vi "PP Template (UserEvent).vi"() -> ()   [LabVIEW 2011, in "Messenging.lvlib" / "PP Template (UserEvent).lvclass"]
uses:
  PP Template (UserEvent).lvclass
  Interprocess Messenger/TextVarientMessage/MSG.lvclass
  Parallel Process.lvclass
  Interprocess Messenger/EventMessenger/EventMessenger.lvclass
  ObserverRegister/ObserverRegistry.lvclass
  Interprocess Messenger/TextVarientMessage/Write (no data).vi
  Interprocess Messenger/ErrorMessage/Write ErrorMessage.vi
  Interprocess Messenger/ErrorMessage/ErrorMessage.lvclass
  Interprocess Messenger/TextVarientMessage/Write VarMessage.vi
  Interprocess Messenger/VarMessage/VarMessage.lvclass
panel:
  out "date/time string":string
  in  "Startup Message":refnum<class "MSG.lvclass">
  # "EventMesssenger based"
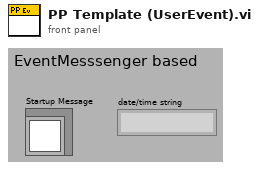
[diagram p1: front panel]
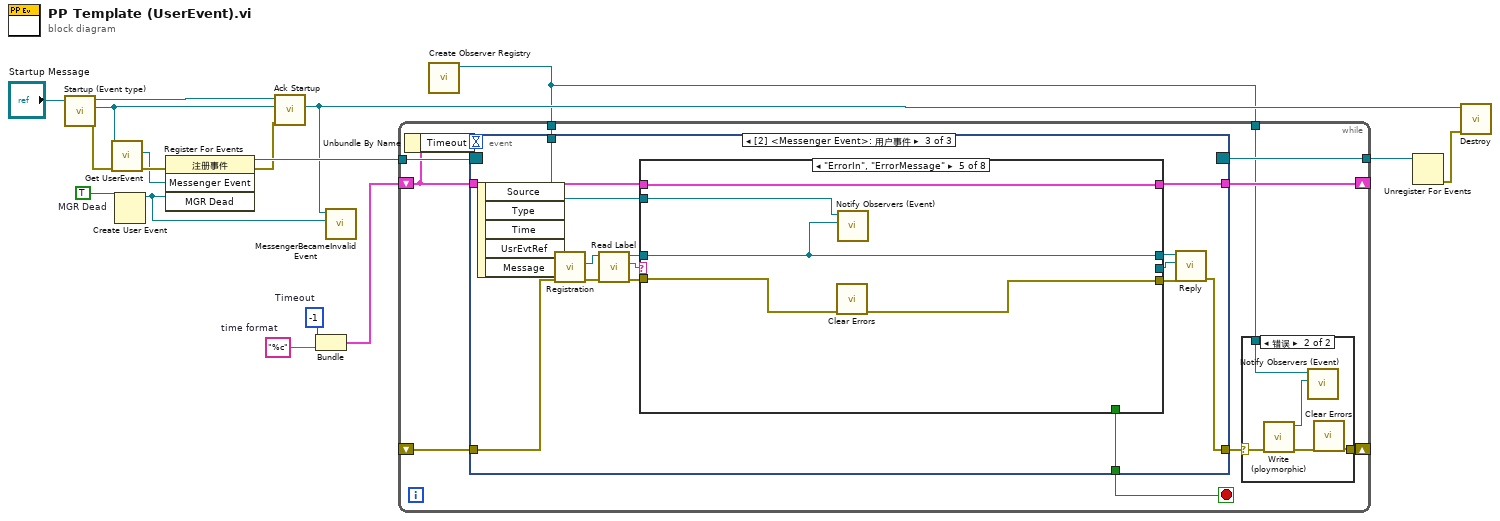
[diagram p0: block diagram]
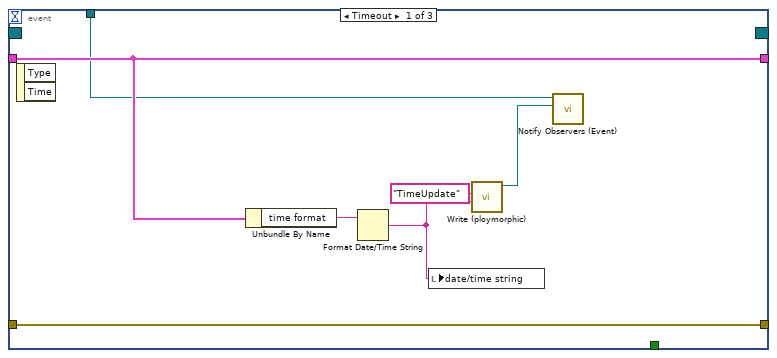
[diagram p3: hidden frame]
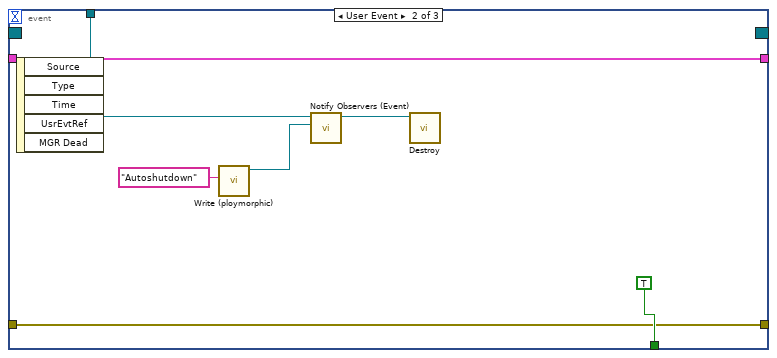
[diagram p4: hidden frame]
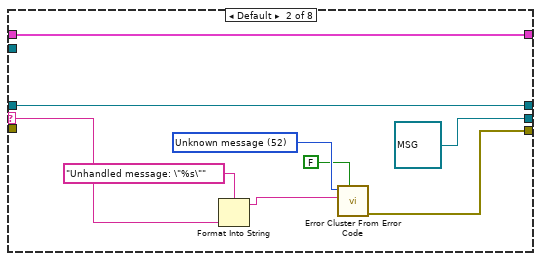
[diagram p6: hidden frame]
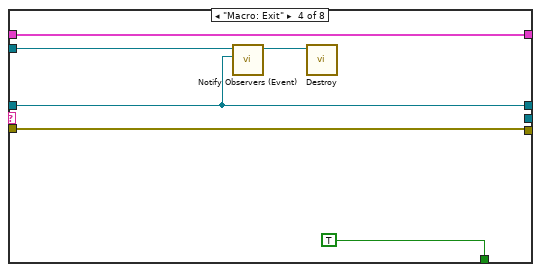
[diagram p8: hidden frame]
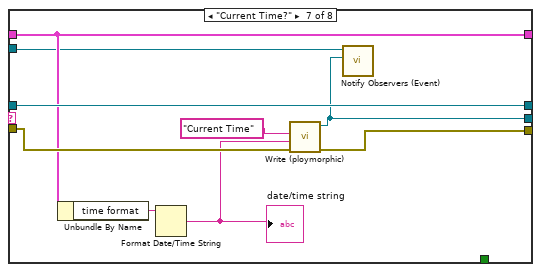
[diagram p10: hidden frame]
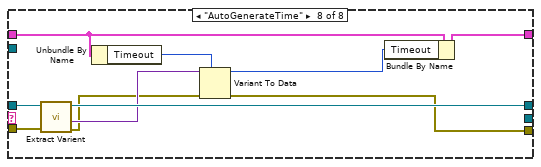
[diagram p11: hidden frame]
diagram:
  w2 = "%c"  # time format
  w6 = TRUE  # MGR Dead
  w9 = -1  # Timeout
  n1 = call "Startup (Event type).vi"("Startup Message"="Startup Message") -> ("error out"=w15:errorcluster, "Command Messenger out"=w17:refnum<class "EventMessenger.lvclass">, "Starup Message"=w16:refnum<class "MSG.lvclass">)  [unwired: 2 in, 6 out]
  n2 = call-dynamic "Get UserEvent.vi"("error in"=w15, "EventMessenger"=w17) -> ("error out"=w13:errorcluster, "Messenger Event"=w7:refnum<user-event>)  [unwired: 8 out]
  n3 = Create User Event(user event datatype=w6) -> (user event=w4:refnum<user-event>)  [unwired: 1 in, 1 out]
  n4 = register-events(error in=w13, w7, w4) -> (reference out=w12:refnum<event-registration>, error out=w5:errorcluster)  [unwired: 1 in]
  n5 = call "Ack Startup.vi"("error in"=w5, "Command Messenger"=w17, "Starup Message"=w16) -> ("Command Messenger"=w3:refnum<class "EventMessenger.lvclass">)  [unwired: 3 in, 5 out]
  n6 = Bundle("Timeout"=w9, "time format"=w2) -> (w8:cluster{"Timeout":i32, "time format":string})  [unwired: 1 out]
  n7 = call "MessengerBecameInvalid Event.vi"("MGR became Invalid"=w4, "Messenger"=w3) -> ()  [unwired: 1 in, 9 out]
  n8 = call "Create Observer Registry.vi"() -> ("ObsReg"=w1:refnum<class "ObserverRegistry.lvclass">)  [unwired: 1 in, 10 out]
  n9 = while {
    tunnel: w12 -> [w28]
    tunnel: [w27] -> w11
    shift-right: [w21] -> _
    shift-left: w8 -> [w25]
    shift-right: [w20] -> _
    shift-left: _ -> [w23]
    tunnel: w1 -> [w19]
    tunnel: w1 -> [w18]
    stop <- w26 stop-if-true
    n10 = Unbundle By Name(w25) -> ("Timeout"=w24:i32)
    n11 = event shown="[2] <Messenger Event>: 用户事件" {
      selector: w28 -> [_ _ _]
      dyn-events: [_ _ _] -> w27
      timeout: w24 -> [_ _ _]
      tunnel: [_ TRUE ("Shutdown if Receiver Dead") w54] -> w26
      tunnel: w25 -> [w37 w48 w56]
      tunnel: [w37 w48 w55] -> w21
      tunnel: [w35 w46 w53] -> w22
      tunnel: w23 -> [w35 w46 w52]
      tunnel: w19 -> [w36 w45 w49]
      event Timeout {
        n12 = event-data() -> ()  [unwired: 3 out]
        n13 = Unbundle By Name(w37) -> ("time format"=w41:string)
        n14 = Format Date/Time String(time format string (%c)=w41) -> (date/time string=w38:string)  [unwired: 2 out]
        n15 = local write "date/time string"(w38) -> ()
        n16 = call-poly "Write (ploymorphic).vi"("Varient"=w38, "Label"="TimeUpdate") -> ("Message"=w39:refnum<class "VarMessage.lvclass">)  [unwired: 1 in, 8 out]
        n17 = call "Notify Observers (Event).vi"("Message"=w39, "ObserverRegistry in"=w36) -> ()  [unwired: 1 in, 9 out]
      }
      event User Event {
        n18 = event-data() -> ()  [unwired: 6 out]
        n19 = call-poly "Write (ploymorphic).vi"("Label"="Autoshutdown") -> ("Message"=w42:refnum<class "MSG.lvclass">)  [unwired: 1 in, 9 out]
        n20 = call "Notify Observers (Event).vi"("Message"=w42, "ObserverRegistry in"=w45) -> ("ObserverRegistry out"=w44:refnum<class "ObserverRegistry.lvclass">)  [unwired: 1 in, 8 out]
        n21 = call "Destroy.vi"("ObserverRegistry.lvclass in"=w44) -> ()  [unwired: 1 in, 10 out]
      }
      event User Event {
        n22 = event-data() -> ("Message"=w51:refnum<class "MSG.lvclass">)  [unwired: 5 out]
        n23 = call "Registration.vi"("Message"=w51, "ObserverRegistry in"=w49) -> ("Message (Register Commands filtered out)"=w50:refnum<class "MSG.lvclass">)  [unwired: 1 in, 8 out]
        n24 = call-dynamic "Read Label.vi"("error in (no error)"=w52, "Message"=w50) -> ("error out"=w58:errorcluster, "Label"=w57:string, "Message"=w59:refnum<class "MSG.lvclass">)  [unwired: 7 out]
        n25 = case shown="\"ErrorIn\", \"ErrorMessage\"" w57 {
          selector: w57 -> [_ w74 _ _ _ _ _ _]
          tunnel: w58 -> [w65 _ w77 w79 w85 w91 w99 w108]
          tunnel: w59 -> [w64 w68 w76 w80 w87 w90 w100 w110]
          tunnel: [w65 w69 w77 w79 w84 w91 w98 w101] -> w62
          tunnel: [w64 w68 w76 w80 w87 w90 w100 w109] -> w60
          tunnel: [_ refnum<class "MSG.lvclass"> refnum ("Messenging.lvlib:Interprocess Message") _ _ _ _ w94 _] -> w61
          tunnel: [_ _ _ TRUE _ _ _ _] -> w54
          tunnel: [w63 w66 w75 w83 w88 w89 w97 w104] -> w55
          tunnel: w56 -> [w63 w66 w75 w83 w88 w89 w97 w106]
          tunnel: w49 -> [_ _ _ w78 w86 _ w93 _]
          frame "------- Core ----------" {
            # "Core Cases for template"
          }
          frame Default {
            w71 = 52 items=["No error", "Argument error", "Memory is full", "Out of zone", "End of file", "File already open", "Generic file I/O error", "File not found", "File permission error", "Disk is full", "Duplicate path", "Too many files open", "System feature not enabled", "Resource file not found", "Cannot add resource", "Resource not found", "Image not found", "Image memory error", "Pen does not exist", "Config type invalid", "Config token not found", "Config parse error", "Config memory error", "Bad external code format", "Bad external code offset", "External code not present", "Null window", "Destroy window error", "Null menu", "Print aborted", "Bad print record", "Print driver error", "Windows error during printing", "Memory error during printing", "Print dialog error", "Generic print error", "Invalid device refnum", "Device not found", "Device parameter error", "Device unit error", "Cannot open device", "Device call aborted", "Generic error", "Cancelled by user", "Object ID too low", "Object ID too high", "Object not in heap", "Unknown heap", "Unknown object (invalid DefProc)", "Unknown object (DefProc not in table)", "Message out of range", "Invalid (null) method", "Unknown message", "Manager call not supported", "Bad address", "Network operation in progress", "Network operation timed out", "Connection is busy", "Network attribute not supported", "Network error", "Address in use", "System out of memory", "Connection aborted", "Connection refused", "Not connected", "Already connected", "Connection closed", "Initialization error (interapplication manager)", "Bad occurrence", "Wait on unbound occurrence handler", "Occurrence queue overflow", "Datalog type conflict", "Unused", "Unrecognized type (interapplication manager)", "Memory corrupt", "Failed to make temporary DLL", "Old CIN version", "Drag socket not found", "Failed to load drop-object", "Failed to register OLE object", "Failed to release OLE object", "Format specifier type mismatch", "Unknown format specifier", "Too few format specifiers", "Too many format specifiers", "Scan failed", "Newer CIN version", "Error converting to variant", "Runtime menu error", "Password tampered", "Variant attribute not found", "Incompatible variant data type", "Event data is not available", "Event Store is not present", "Occurrence is not found", "Event Queue is not created", "Event info is not available", "Refnum passed is NULL", "Error retrieving Class GUID", "Error retrieving CoClass GUID", "Error retrieving TypeLib GUID.", "Bad built application magic bytes.", "Specific driver is different from the specific driver associated with the Logical Name.", "There is no session opened to the class driver.", "Max Error", "MAX - Error with config objects", "MAX - Error loading configuration", "MAX - Group not supported"]
            n26 = Format Into String(format string="Unhandled message: \"%s\"", w74) -> (resulting string=w72:string)  [unwired: 2 in, 1 out]
            n27 = call <vilib>:"Error Cluster From Error Code.vi"("show call chain? (False)"=FALSE, "error message (\"\")"=w72, "error code (0)"=w71) -> ("error out"=w69:errorcluster)  [unwired: 1 in, 5 out]
          }
          frame "MSG" {
            # "NULL message --> do nothing"
          }
          frame "Macro: Exit" {
            n28 = call "Notify Observers (Event).vi"("Message"=w80, "ObserverRegistry in"=w78) -> ("ObserverRegistry out"=w81:refnum<class "ObserverRegistry.lvclass">)  [unwired: 1 in, 8 out]
            n29 = call "Destroy.vi"("ObserverRegistry.lvclass in"=w81) -> ()  [unwired: 1 in, 10 out]
          }
          frame "ErrorIn", "ErrorMessage" {
            n30 = call <vilib>:"Clear Errors.vi"("error in (no error)"=w85) -> ("error out"=w84:errorcluster)  [unwired: 6 out]
            n31 = call "Notify Observers (Event).vi"("Message"=w87, "ObserverRegistry in"=w86) -> ()  [unwired: 1 in, 9 out]
          }
          frame "-------- Example --------" {
            # "Example Cases: replace when using template"
          }
          frame "Current Time?" {
            n32 = Unbundle By Name(w97) -> ("time format"=w96:string)
            n33 = Format Date/Time String(time format string (%c)=w96) -> (date/time string=w92:string)  [unwired: 2 out]
            "date/time string" <- w92
            n34 = call-poly "Write (ploymorphic).vi"("error in (no error)"=w99, "Varient"=w92, "Label"="Current Time") -> ("error out"=w98:errorcluster, "Message"=w94:refnum<class "VarMessage.lvclass">)  [unwired: 7 out]
            n35 = call "Notify Observers (Event).vi"("Message"=w94, "ObserverRegistry in"=w93) -> ()  [unwired: 1 in, 9 out]
          }
          frame "AutoGenerateTime" {
            n36 = call-dynamic "Extract Varient.vi"("error in (no error)"=w108, "Message"=w110) -> ("error out"=w102:errorcluster, "Varient"=w107:variant, "Message"=w109:refnum<class "MSG.lvclass">)  [unwired: 1 in, 6 out]
            n37 = Unbundle By Name(w106) -> ("Timeout"=w105:i32)
            n38 = Variant To Data(error in=w102, type=w105, Variant=w107) -> (data=w103:i32, error out=w101:errorcluster)
            n39 = Bundle By Name(cluster=w106, "Timeout"=w103) -> (w104:cluster{"Timeout":i32, "time format":string})
          }
        }
        n40 = call-dynamic "Reply.vi"("error in (no error)"=w62, "Reply"=w61, "Message to Reply to"=w60) -> ("error out"=w53:errorcluster)  [unwired: 8 out]
      }
    }
    n41 = case shown="错误" w22 {
      selector: w22 -> [w29 w34]
      tunnel: [w29 w33] -> w20
      tunnel: w18 -> [_ w30]
      frame No Error {
      }
      frame Error {
        n42 = call-poly "Write (ploymorphic).vi"("error (to be sent)"=w34) -> ("error out"=w32:errorcluster, "Message"=w31:refnum<class "ErrorMessage.lvclass">)  [unwired: 1 in, 8 out]
        n43 = call "Notify Observers (Event).vi"("Message"=w31, "ObserverRegistry in"=w30) -> ()  [unwired: 1 in, 9 out]
        n44 = call <vilib>:"Clear Errors.vi"("error in (no error)"=w32) -> ("error out"=w33:errorcluster)  [unwired: 6 out]
      }
    }
  }
  n45 = Unregister For Events(event registration refnum=w11) -> (error out=w10:errorcluster)  [unwired: 1 in]
  n46 = call-dynamic "Destroy.vi"("error in (no error)"=w10, "EventMessenger in"=w3) -> ()  [unwired: 10 out]
